vi "test Verify Scripting Code.vi"(8 "error in":errorcluster, 11 "Test Case In":refnum<class "LUnit Extensions Tests.lvclass">) -> (0 "error out":errorcluster, 3 "Test Case Out":refnum<class "LUnit Extensions Tests.lvclass">)   [LabVIEW 2020, in "LUnit Extensions Tests.lvclass"]
uses:
  LUnit Extensions Tests.lvclass
  LUnit Extensions Tests.lvclass/LUnit Extensions Tests.ctl
  Source/Extensions/LUnit.Extension/LUnit.Extension.lvlib
  C:/Program Files/National Instruments/LabVIEW 2020/vi.lib/Astemes/LUnit/Test Case.lvclass
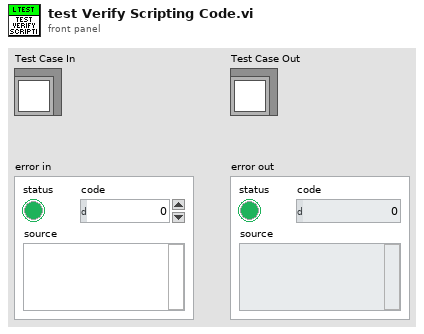
[diagram p1: front panel]
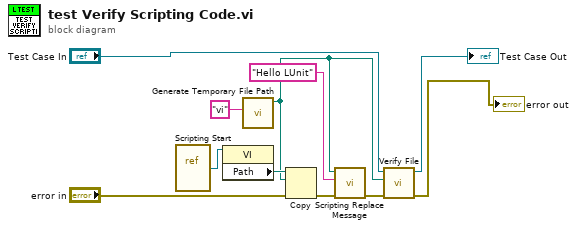
[diagram p0: block diagram]
diagram:
  n1 = vi-ref "Scripting Start.vi"() -> (w5:refnum<vi>)
  n2 = property on="Property Node" class="VI"(reference=w5) -> ("Path"=w2:path)  [unwired: 1 in, 2 out]
  n3 = call <vilib>:"Generate Temporary File Path.vi"("Temporary File Extension (tmp)"="vi") -> ("Unique Temporary File Path"=w1:path)  [unwired: 9 in, 1 out]
  n4 = Copy(8:"error in", 10:w1, 11:w2) -> (0:w9:errorcluster)  [unwired: 2 in, 2 out]
  n5 = call "Scripting Replace Message.vi"("error in"=w9, "New Message"="Hello LUnit", "Path"=w1) -> ("error out"=w8:errorcluster)  [unwired: 8 in]
  n6 = call "Verify File.vi"("error in"=w8, "path to file"=w1, "LUnit Test Case In"="Test Case In") -> ("error out"=→"error out":errorcluster, "LUnit Test Case Out"=→"Test Case Out":refnum<class "LUnit Extensions Tests.lvclass">)  [unwired: 7 in]
